vi "server_tcp.vi"() -> ()   [LabVIEW 2016]
uses:
  lab4/genetrator/Control 4.ctl
  lab4/genetrator/Control 5.ctl
  lab4/genetrator/Control 6.ctl
  lab4/genetrator/Control 2.ctl
  lab4/genetrator/Control 1.ctl
panel:
  in  "krok [ms]":T1=100.0 caption="Frequency"
  in  "Clear":bool
  out "wynik dzialania":cluster{"Y":dbl[], "Y":dbl[]}[](graph)
  in  "czestotl [Hz]":T1=1.0 caption="Frequency"
  in  "amplituda":T2=10.0 caption="Frequency"
  in  "dzialanie":T3 items=["+", "-", "*", "/", ""]
  in  "z jakim?":T4 items=["sin", "square", "sawtooth", "noise"]
  in  "jaki sygna³?":T5 items=["sin", "square", "sawtooth", "noise"]
  in  "Stop":bool
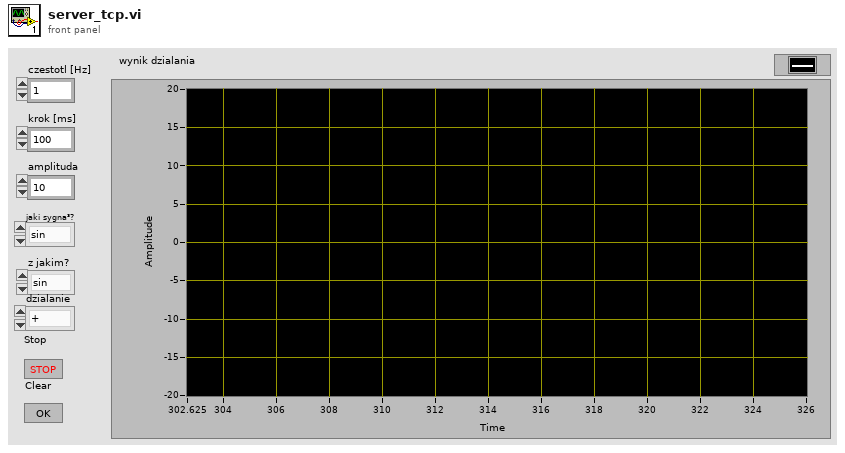
[diagram p1: front panel]
types:
  T1 = typedef "Control 1.ctl" = dbl
  T2 = typedef "Control 2.ctl" = dbl
  T3 = typedef "Control 6.ctl" = u16
  T4 = typedef "Control 5.ctl" = u16
  T5 = typedef "Control 4.ctl" = u16
  T6 = typedef "Control 3.ctl" = dbl
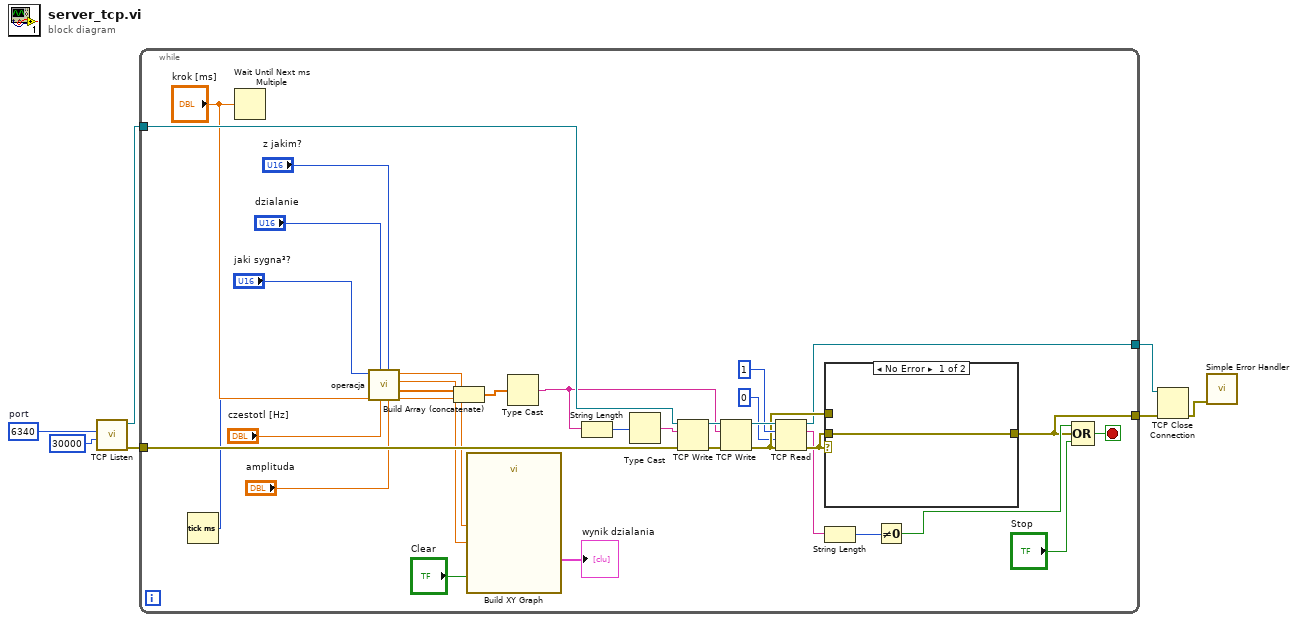
[diagram p0: block diagram]
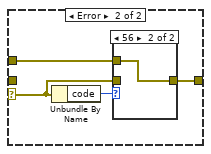
[diagram p2: hidden frame]
diagram:
  w7 = u16 6340  # port
  n1 = call <vilib>:"TCP Listen.vi"("timeout ms (wait forever: -1)"=30000, "port"=w7) -> ("error out"=w6:errorcluster, "connection ID"=w5:refnum<k5>)  [unwired: 5 in, 3 out]
  n2 = while {
    tunnel: w6 -> [w39]
    tunnel: w5 -> [w38]
    tunnel: [w22] -> w4
    tunnel: [w21] -> w3
    stop <- w25 stop-if-true
    n3 = Tick Count (ms)() -> (millisecond timer value=w8:u32)
    n4 = Wait Until Next ms Multiple(millisecond multiple="krok [ms]") -> ()  [unwired: 1 out]
    n5 = call "operacja.vi"("amplituda in"="amplituda", "z jakim?"="z jakim?", "czestotl [Hz]"="czestotl [Hz]", "dzialanie"="dzialanie", "millisecond timer value"=w8, "jaki sygna³?"="jaki sygna³?") -> ("Array"=w12:T2[], "amplituda out"=w17:T2, "x pocz out"=w18:T6)  [unwired: 3 in]
    n6 = Build Array (concatenate)(w12, "krok [ms]") -> (w11:T1[])
    n7 = call "Build XY Graph"("Reset"="Clear", "Y Input"=w17, "X Input"=w18) -> ("XY Graph"=→"wynik dzialania":cluster{"Y":dbl[], "Y":dbl[]}[])  [unwired: 7 in, 1 out]
    n8 = Type Cast(x=w11) -> (*(type *) &x=w10:string)  [unwired: 1 out]
    n9 = String Length(string=w10) -> (length=w15:i32)
    n10 = Type Cast(x=w15) -> (*(type *) &x=w14:string)  [unwired: 1 out]
    n11 = TCP Write(connection ID=w38, data in=w14, error in (no error)=w39) -> (connection ID out=w33:refnum<k5>, error out=w32:errorcluster)  [unwired: 2 out]
    n12 = TCP Write(connection ID=w33, data in=w10, error in (no error)=w32) -> (connection ID out=w31:refnum<k5>, error out=w28:errorcluster)  [unwired: 2 out]
    n13 = TCP Read(connection ID=w31, bytes to read=1, error in (no error)=w28, 9:0) -> (connection ID out=w21:refnum<k5>, data out=w26:string, error out=w29:errorcluster)  [unwired: 1 out]
    n14 = case shown="No Error" w29 {
      selector: w29 -> [_ w43]
      tunnel: w29 -> [w40 _]
      tunnel: [w40 w42] -> w22
      tunnel: w28 -> [_ w41]
      frame No Error {
      }
      frame Error {
        n15 = Unbundle By Name(w43) -> ("code"=w44:i32)
        n16 = case shown="56" w44 {
          tunnel: w43 -> [w45 _]
          tunnel: [w45 w46] -> w42
          tunnel: w41 -> [_ w46]
          frame Default {
          }
          frame 56 {
          }
        }
      }
    }
    n17 = String Length(string=w26) -> (length=w27:i32)
    n18 = Not Equal To 0?(x=w27) -> (x != 0?=w23:bool)
    n19 = Compound Arithmetic op=OR(w23, w22, "Stop") -> (w25:bool)
  }
  n20 = TCP Close Connection(connection ID=w3, error in (no error)=w4) -> (error out=w1:errorcluster)  [unwired: 2 out]
  n21 = call <vilib>:"Simple Error Handler.vi"("error in (no error)"=w1) -> ()  [unwired: 4 in, 5 out]
